vi "Tosca-Globals.vi"() -> ()   [LabVIEW 2020]
uses:
  Digital Input VIs/Tosca-Input Event.ctl
  Digital Input VIs/Tosca-Input Criterion.ctl
  epl-vi-lib/Utility VIs/Type Defs/Logic State.ctl
  Typedefs/Tosca-Accumulator.ctl
panel:
  in  "Version":string="4.15.1"
  in  "Input Events":T1[](array[typedef])
  out "Rig":string="Tosca"
  in  "datafile":path
  in  "Cal folder":path=path "C:/Data/Tosca/Calibration Files"
  out "Config":string="Tosca"
  out "Flags":i32[](array[numeric])
  out "DI dt":i32
  out "Headway (%)":dbl
  out "Nerror":i32
  out "Max errors":i32
  in  "Masker Level":dbl
  # "Masker"
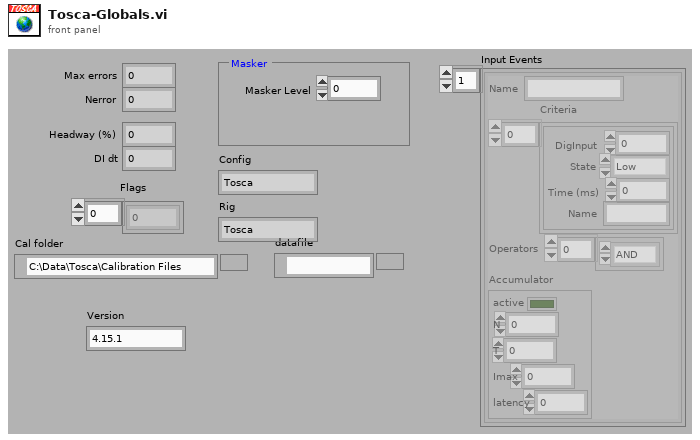
[diagram p1: front panel]
types:
  T1 = typedef "Tosca-Input Event.ctl" = cluster{"Name":string, "Criteria":T2[], "Operators":enum16{"AND", "OR"}[], "Accumulator":T4}
  T2 = typedef "Tosca-Input Criterion.ctl" = cluster{"DigInput":i32, "State":T3, "Time (ms)":i32, "Name":string}
  T3 = typedef "Logic State.ctl" = enum16{"Low", "High", "Rising", "Falling"}
  T4 = typedef "Tosca-Accumulator.ctl" = cluster{"active":bool, "N":i32, "T":dbl, "Imax":dbl, "latency":dbl}
diagram:
